vi "camera_calibration.vi"() -> ()   [LabVIEW 2021]
doc: "This example demonstrates how to call a Python function and pass integers as arguments. It uses a python function to compute the sum of two integers."
uses:
  Program Files (x86)/National Instruments/LabVIEW 2021/examples/Connectivity/Python/support/PythonVersionsEnum.ctl
panel:
  out "error out":errorcluster
  in  "error in (no error)":errorcluster
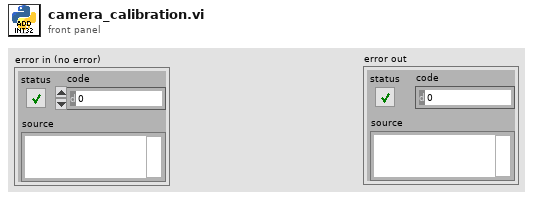
[diagram p1: front panel]
types:
  T1 = typedef "PythonVersionsEnum.ctl" = enum16{"3.6", "3.7", "3.8", "3.9"}
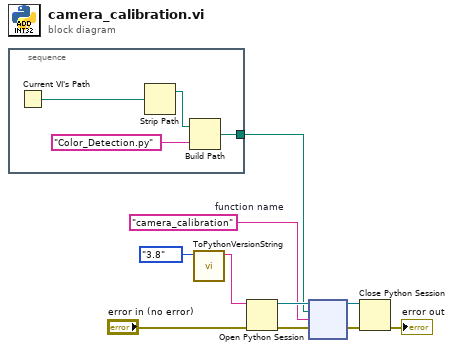
[diagram p0: block diagram]
diagram:
  w6 = "camera_calibration"  # function name
  n1 = stacked-sequence {
    tunnel: [w14] -> w7
    frame #0 {
      n2 = Current VI's Path() -> (path=w11:path)
      n3 = Strip Path(path=w11) -> (stripped path=w12:path)  [unwired: 1 out]
      n4 = Build Path(base path=w12, name or relative path="Color_Detection.py") -> (appended path=w14:path)
    }
  }
  n5 = call "ToPythonVersionString.vi"("python version"=PythonVersionsEnum."3.8") -> ("python version string"=w2:string)  [unwired: 10 in]
  n6 = Open Python Session(python version=w2, 3:"error in (no error)") -> (session out=w9:refnum<k35>, error out=w8:errorcluster)  [unwired: 1 in]
  n7 = node(w9, w7, w6, w8) -> (w5:refnum<k35>, w4:errorcluster)  [unwired: 2 in, 2 out]
  n8 = Close Python Session(session in=w5, error in=w4) -> (11:→"error out":errorcluster)
